vi "Add Message to Remote Terminal.vi"(4 "create timestamp channel":bool, 5 "remote terminal":T2, 6 "parameters":T5(array[cluster]), 7 "number of words":u16, 8 "error in":errorcluster, 9 "direction":T6, 10 "name":string, 11 "port in":T1 format="%.0x") -> (0 "error out":errorcluster, 2 "message":T1=18446744073709551615 format="%.0x", 3 "port out":T1 format="%.0x")   [LabVIEW 2020, in "Ballard MIL-STD-1553 Scripting.lvlib"]
uses:
  Ballard MIL-STD-1553 Scripting.lvlib
  Shared/Direction.ctl
  Shared/Parameter Definition.ctl
  Shared/Terminal Endpoint.ctl
  Shared/Address.ctl
  <vilib>/NI VeriStand/Custom Device API/Custom Device Item Ref.ctl
  <vilib>/NI VeriStand/Custom Device API/Custom Device API.lvlib
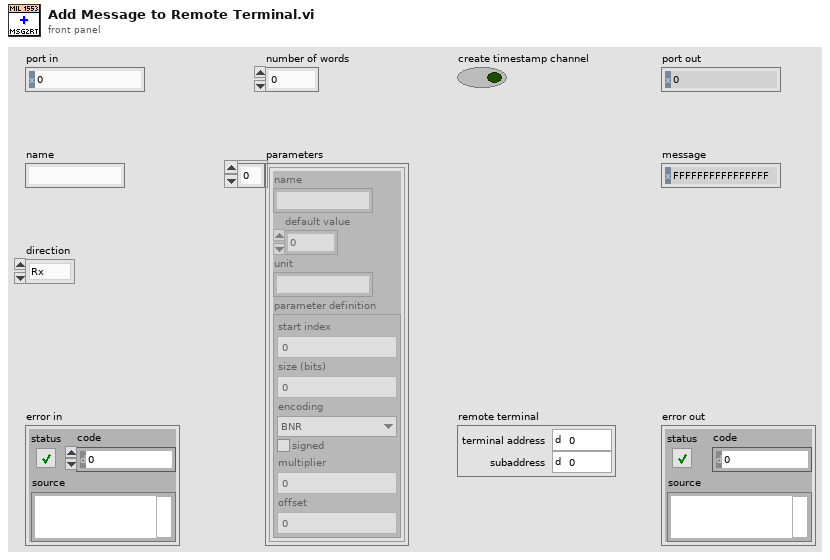
[diagram p1: front panel]
types:
  T1 = typedef "Custom Device API.lvlib/Custom Device Item Ref.ctl" = u64
  T2 = typedef "Terminal Endpoint.ctl" = cluster{"terminal address":T3, "subaddress":T3}
  T3 = typedef "Address.ctl" = u16
  T4 = typedef "Parameter Definition.ctl" = cluster{"start index":i32, "size (bits)":i32, "encoding":enum16{"BNR", "BCD", "Discrete"}, "signed":bool, "multiplier":dbl, "offset":dbl}
  T5 = cluster{"name":string, "default value":dbl, "unit":string, "parameter definition":T4}[]
  T6 = typedef "Direction.ctl" = enum16{"Rx", "Tx"}
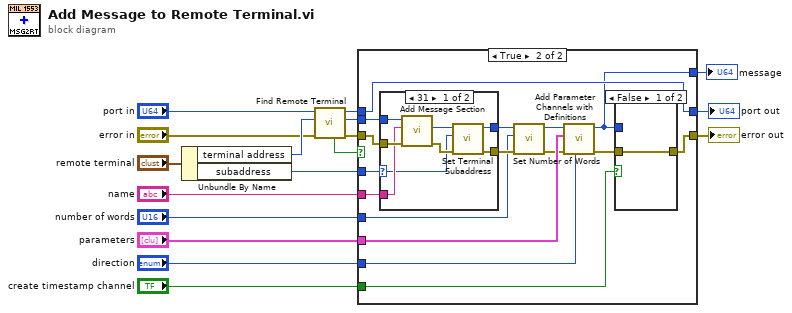
[diagram p0: block diagram]
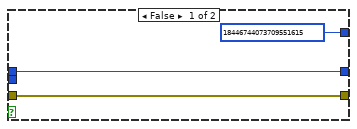
[diagram p2: hidden frame]
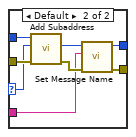
[diagram p3: hidden frame]
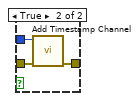
[diagram p4: hidden frame]
diagram:
  n1 = Unbundle By Name("remote terminal") -> ("terminal address"=w10:T3, "subaddress"=w12:T3)
  n2 = call "Find Remote Terminal.vi"("error in"="error in", "terminal address"=w10, "port in"="port in") -> ("error out"=w2:errorcluster, "remote terminal"=w3:T1, "port out"=w4:T1, "found?"=w5:bool)  [unwired: 5 in]
  n3 = case shown="True" w5 {
    tunnel: w4 -> [w20 w22]
    tunnel: w3 -> [_ w35]
    tunnel: w2 -> [w19 w36]
    tunnel: [w19 w25] -> w9
    tunnel: [w20 w22] -> w8
    tunnel: w12 -> [_ w34]
    tunnel: "number of words" -> [_ w27]
    tunnel: "parameters" -> [_ w33]
    tunnel: "name" -> [_ w28]
    tunnel: "direction" -> [_ w26]
    tunnel: "create timestamp channel" -> [_ w23]
    tunnel: [T1 18446744073709551615 ("message out") w21] -> w1
    frame False {
    }
    frame True {
      n4 = case shown="31" w34 {
        selector: w34 -> [w37 w50]
        tunnel: w36 -> [w43 w52]
        tunnel: w35 -> [w44 w51]
        tunnel: [w40 w47] -> w32
        tunnel: [w38 w46] -> w31
        tunnel: w28 -> [w42 w45]
        frame 31 {
          n5 = call "Add Message Section.vi"("error in"=w43, "message name"=w42, "bus controller in"=w44) -> ("error out"=w39:errorcluster, "message"=w41:T1)  [unwired: 6 in, 1 out]
          n6 = call "Set Terminal Subaddress.vi"("error in"=w39, "subaddress"=w37, "subaddress in"=w41) -> ("error out"=w38:errorcluster, "subaddress out"=w40:T1)  [unwired: 7 in]
        }
        frame Default {
          n7 = call "Add Subaddress.vi"("error in"=w52, "subaddress"=w50, "remote terminal in"=w51) -> ("error out"=w48:errorcluster, "subaddress ref"=w49:T1)  [unwired: 6 in, 1 out]
          n8 = call "Set Message Name.vi"("error in"=w48, "message name"=w45, "message in"=w49) -> ("error out"=w46:errorcluster, "message out"=w47:T1)  [unwired: 7 in]
        }
      }
      n9 = call "Set Number of Words.vi"("error in"=w31, "number of words"=w27, "message in"=w32) -> ("error out"=w29:errorcluster, "message out"=w30:T1)  [unwired: 7 in]
      n10 = call "Add Parameter Channels with Definitions.vi"("direction"=w26, "error in"=w29, "parameters"=w33, "message in"=w30) -> ("error out"=w24:errorcluster, "message out"=w21:T1)  [unwired: 6 in]
      n11 = case shown="False" w23 {
        tunnel: w24 -> [w53 w56]
        tunnel: w21 -> [_ w55]
        tunnel: [w53 w54] -> w25
        frame False {
        }
        frame True {
          n12 = call "Add Timestamp Channel.vi"("error in"=w56, "message section"=w55) -> ("error out"=w54:errorcluster)  [unwired: 8 in, 1 out]
        }
      }
    }
  }
  "error out" <- w9
  "port out" <- w8
  "message" <- w1
